vi "Read XML.vi"() -> (0 "error out":errorcluster caption="错误输出", 3 "值":T1)   [LabVIEW 2016, in "Alarm interface.lvlib"]
uses:
  Alarm interface.lvlib
  <vilib>/Utility/xml.llb/Read From XML File(string).vi
panel:
  in  "一级报警":i32(listbox)
  out "project":T2
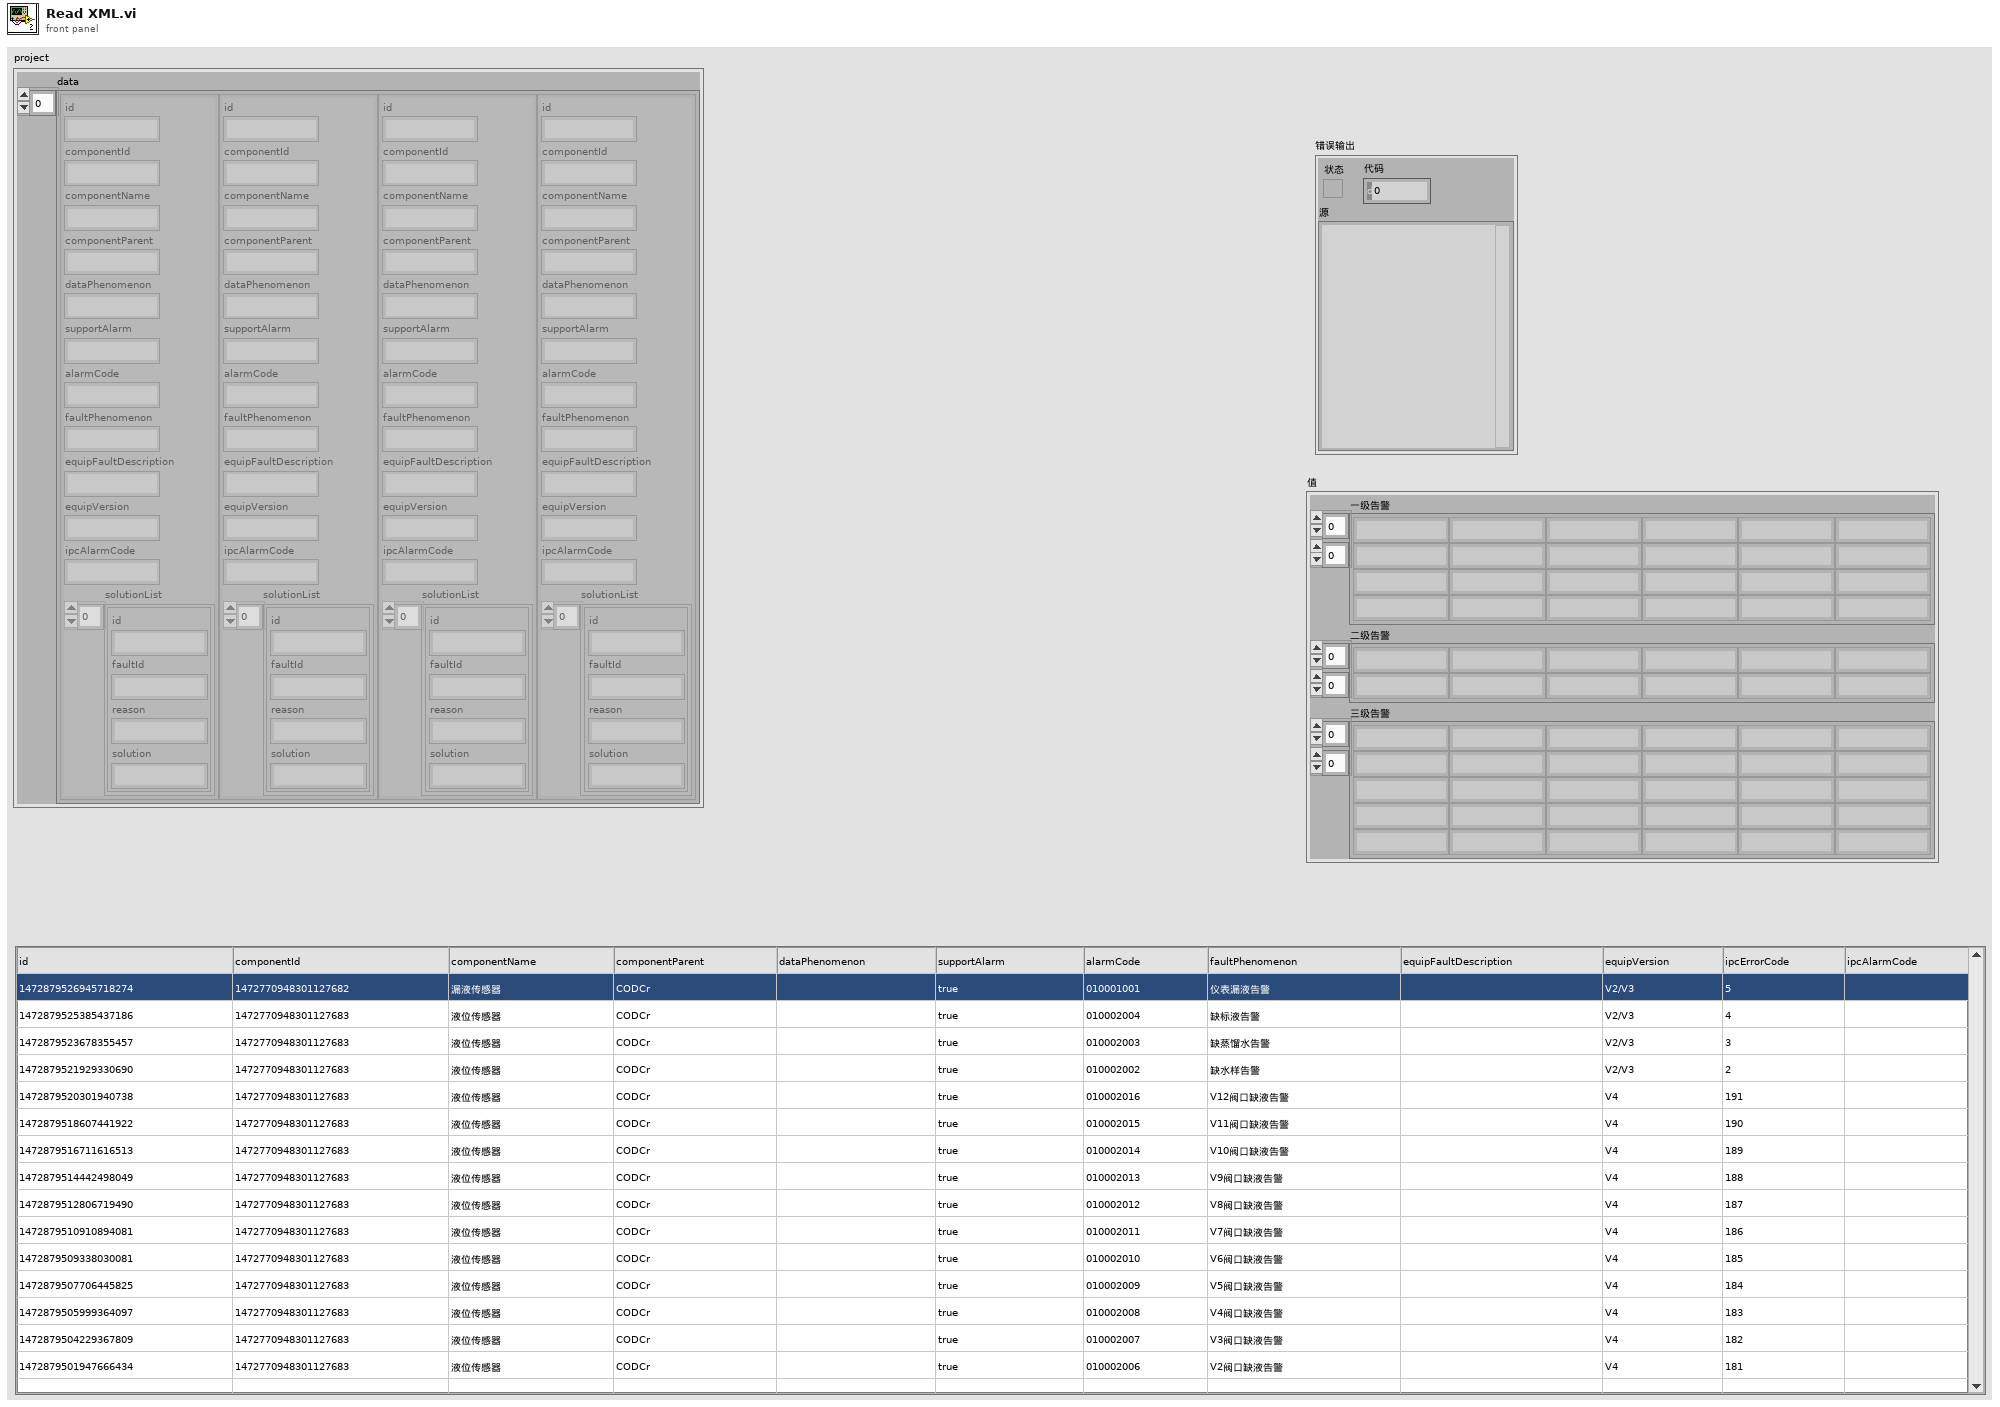
[diagram p1: front panel]
types:
  T1 = cluster{"一级告警":string[][], "二级告警":string[][], "三级告警":string[][]}
  T2 = cluster{"data":cluster{"id":string, "componentId":string, "componentName":string, "componentParent":string, "dataPhenomenon":string, "supportAlarm":string, "alarmCode":string, "faultPhenomenon":string, "equipFaultDescription":string, "equipVersion":string, "ipcAlarmCode":string, "solutionList":cluster{"id":string, "faultId":string, "reason":string, "solution":string}[]}[]}
  T3 = cluster{"id":string, "componentId":string, "componentName":string, "componentParent":string, "dataPhenomenon":string, "supportAlarm":string, "alarmCode":string, "faultPhenomenon":string, "equipFaultDescription":string, "equipVersion":string, "ipcAlarmCode":string, "solutionList":cluster{"id":string, "faultId":string, "reason":string, "solution":string}[]}[]
  T4 = cluster{"项名":string[][], "项名":string[][], "项名":string[][]}
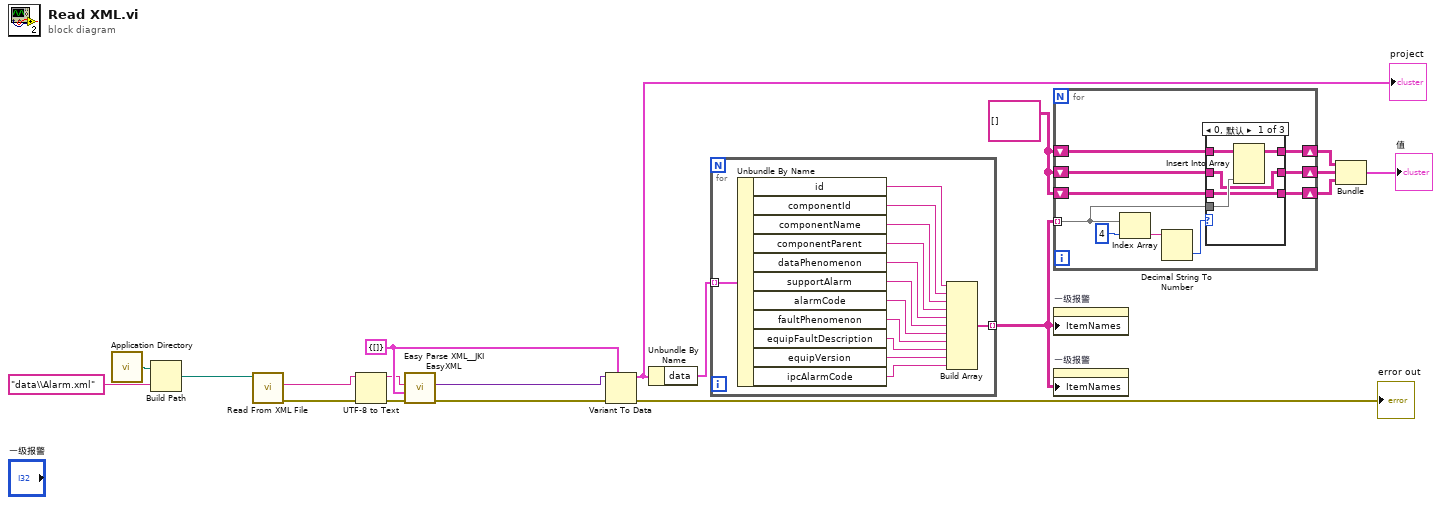
[diagram p0: block diagram]
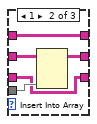
[diagram p2: hidden frame]
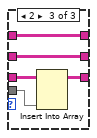
[diagram p3: hidden frame]
diagram:
  w6 = string[][] [] ("项名")
  w13 = T2 {"data"=[]} ("project")
  n1 = call <vilib>:"Application Directory.vi"() -> ("Application Directory"=w19:path)
  n2 = Build Path(base path=w19, name or relative path="data\\Alarm.xml" ("名称或相对路径")) -> (appended path=w17:path)
  n3 = call-poly <vilib>:"Read From XML File.vi"("XML File Path"=w17) -> ("error out"=w10:errorcluster, "XML Elements"=w12:string)  [unwired: 8 in, 1 out]
  n4 = UTF-8 to Text(8:w10, 11:w12) -> (0:w9:errorcluster, 3:w11:string)  [unwired: 1 in]
  n5 = call <vilib>:"Easy Parse XML__JKI EasyXML.vi"("error in (no error)"=w9, "LabVIEW Data (Type)"=w13, "XML String"=w11) -> ("error out"=w14:errorcluster, "LabVIEW Data"=w16:variant)  [unwired: 7 in]
  n6 = Variant To Data(error in=w14, type=w13, Variant=w16) -> (data=w8:T2, error out=→"error out":errorcluster)
  "project" <- w8
  n7 = Unbundle By Name(w8) -> ("data"=w7:T3)
  n8 = for {
    tunnel: w7 -> [w32] mode=indexing
    tunnel: [w21] -> w1 mode=indexing
    n9 = Unbundle By Name(w32) -> ("id"=w31:string, "componentId"=w30:string, "componentName"=w29:string, "componentParent"=w28:string, "dataPhenomenon"=w27:string, "supportAlarm"=w26:string, "alarmCode"=w25:string, "faultPhenomenon"=w24:string, "equipFaultDescription"=w23:string, "equipVersion"=w22:string, "ipcAlarmCode"=w20:string)
    n10 = Build Array(w31, w30, w29, w28, w27, w26, w25, w24, w23, w22, w20) -> (w21:string[])
  }
  n11 = for {
    tunnel: w1 -> [w39] mode=indexing
    shift-right: [w37] -> w5
    shift-left: w6 -> [w38]
    shift-right: [w36] -> w4
    shift-left: w6 -> [w35]
    shift-right: [w33] -> w3
    shift-left: w6 -> [w34]
    n12 = Index Array(array=w39, index=4 ("索引")) -> (element=w41:string)
    n13 = Decimal String To Number(string=w41) -> (number=w40:i32)  [unwired: 2 in, 1 out]
    n14 = case shown="0, 默认" w40 {
      tunnel: w39 -> [w46 w52 w54]
      tunnel: w38 -> [w47 w50 w57]
      tunnel: [w45 w50 w57] -> w37
      tunnel: [w44 w51 w56] -> w36
      tunnel: w35 -> [w44 w49 w56]
      tunnel: w34 -> [w43 w48 w55]
      tunnel: [w43 w48 w53] -> w33
      frame 0, Default {
        n15 = Insert Into Array(array=w47, new element=w46) -> (w45:string[][])  [unwired: 2 in]
      }
      frame 1 {
        n16 = Insert Into Array(array=w49, new element=w52) -> (w51:string[][])  [unwired: 2 in]
      }
      frame 2 {
        n17 = Insert Into Array(array=w55, new element=w54) -> (w53:string[][])  [unwired: 2 in]
      }
    }
  }
  n18 = property on="一级报警" class="MCListbox (严格)"("ItemNames"=w1) -> ()  [unwired: 2 in, 2 out]
  n19 = property on="一级报警" class="MCListbox (严格)"("ItemNames"=w1) -> ()  [unwired: 2 in, 2 out]
  n20 = Bundle("项名"=w5, "项名"=w4, "项名"=w3) -> (→"值":T4)  [unwired: 1 in]
